vi "Transform_STLfile_(SubVI).vi"(8 "error in (no error)":errorcluster, 9 "POSE":dbl[](array[knob])=[0.0, 0.0, 0.0, 0.0, 0.0, 0.0] scale=0.0..90.0, 10 "New Object In":refnum<vi>, 11 "SceneObject In":refnum<vi>) -> (0 "error out":errorcluster, 2 "New Object out":refnum<vi>, 3 "SceneObject Out":refnum<vi>)   [LabVIEW 2015]
uses:
  <vilib>/picture/3D Picture Control/NI_3D Picture Control.lvlib
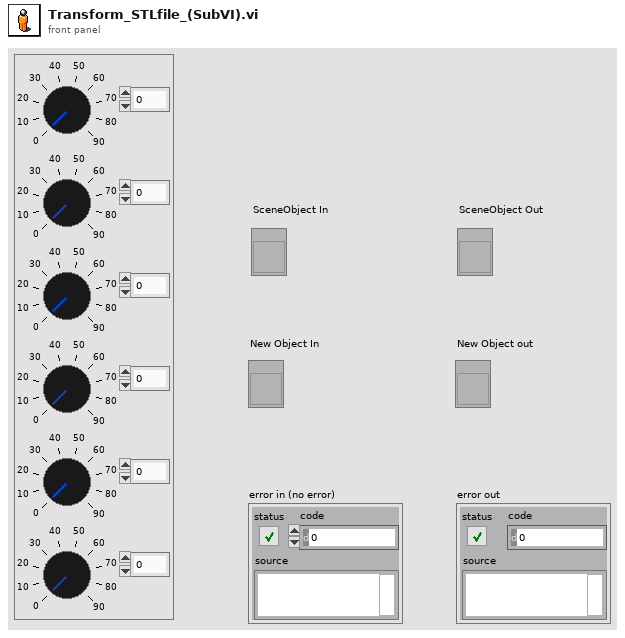
[diagram p1: front panel]
types:
  T1 = cluster{"POSE[0]":dbl, "POSE[1]":dbl, "POSE[2]":dbl, "POSE[3]":dbl, "POSE[4]":dbl, "POSE[5]":dbl}
  T2 = cluster{"POSE[0]":dbl, "POSE[1]":dbl, "POSE[2]":dbl}
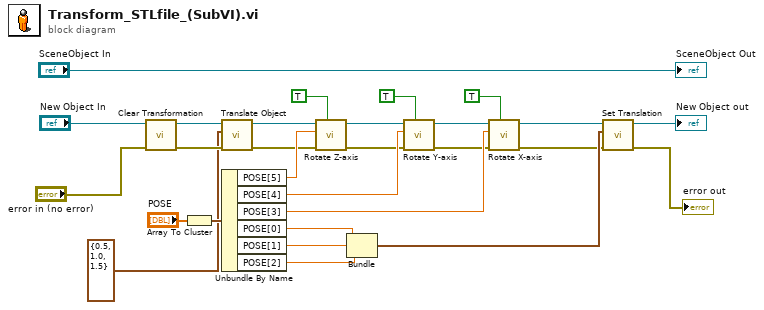
[diagram p0: block diagram]
diagram:
  n1 = call <vilib>:"Clear Transformation.vi"("error in (no error)"="error in (no error)", "Object Refnum In"="New Object In") -> ("error out"=w3:errorcluster, "Object Refnum Out"=w5:refnum<vi>)  [unwired: 8 in]
  n2 = Array To Cluster(array="POSE") -> (cluster=w22:T1)
  n3 = call <vilib>:"Translate Object.vi"("error in (no error)"=w3, "Translation"=cluster{"X":sgl, "Y":sgl, "Z":sgl} {"X"=0.5, "Y"=1.0, "Z"=1.5}, "Scene.Object In"=w5) -> ("error out"=w2:errorcluster, "Scene.Object Out"=w4:refnum<vi>)  [unwired: 7 in]
  n4 = Unbundle By Name(w22) -> ("POSE[5]"=w18:dbl, "POSE[4]"=w19:dbl, "POSE[3]"=w20:dbl, "POSE[0]"=w23:dbl, "POSE[1]"=w24:dbl, "POSE[2]"=w25:dbl)
  n5 = call <vilib>:"Rotate Z-axis.vi"("Relative?"=TRUE, "error in (no error)"=w2, "angle"=w18, "Scene Object In"=w4) -> ("error out"=w9:errorcluster, "Scene Object Out"=w10:refnum<vi>)  [unwired: 6 in]
  n6 = Bundle("POSE[0]"=w23, "POSE[1]"=w24, "POSE[2]"=w25) -> (w26:T2)  [unwired: 1 in]
  n7 = call <vilib>:"Rotate Y-axis.vi"("Relative?"=TRUE, "error in (no error)"=w9, "angle"=w19, "Scene Object In"=w10) -> ("error out"=w12:errorcluster, "Scene Object Out"=w11:refnum<vi>)  [unwired: 6 in]
  n8 = call <vilib>:"Rotate X-axis.vi"("Relative?"=TRUE, "error in (no error)"=w12, "angle"=w20, "Scene Object In"=w11) -> ("error out"=w16:errorcluster, "Scene Object Out"=w17:refnum<vi>)  [unwired: 6 in]
  n9 = call <vilib>:"Set Translation.vi"("error in (no error)"=w16, "Translation"=w26, "Scene Object"=w17) -> ("error out"=→"error out":errorcluster, "Translated Object"=→"New Object out":refnum<vi>)  [unwired: 7 in]
  "SceneObject Out" <- "SceneObject In"
